vi "Get Mac address.vi"(8 "error in (no error)":errorcluster) -> (0 "error out":errorcluster, 3 "MAC address":string)   [LabVIEW 2016]
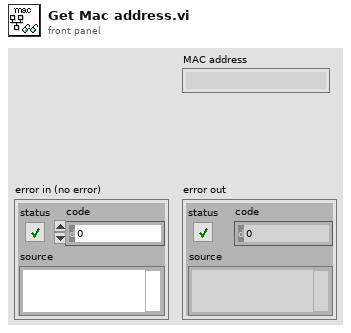
[diagram p1: front panel]
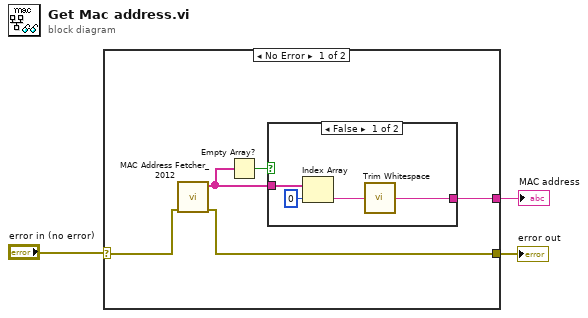
[diagram p0: block diagram]
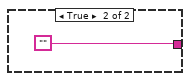
[diagram p2: hidden frame]
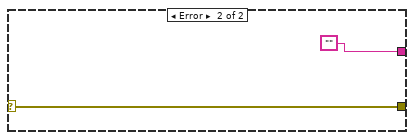
[diagram p3: hidden frame]
diagram:
  n1 = case shown="No Error" "error in (no error)" {
    selector: "error in (no error)" -> [w6 w15]
    tunnel: [w5 w15] -> w2
    tunnel: [w4 ""] -> w1
    frame No Error {
      n2 = call "MAC Address Fetcher_2012.vi"("error in (no error)"=w6) -> ("error out"=w5:errorcluster, "MAC Addresses"=w7:string[])  [unwired: 9 in]
      n3 = Empty Array?(array=w7) -> (empty?=w8:bool)
      n4 = case shown="False" w8 {
        tunnel: w7 -> [w12 _]
        tunnel: [w9 ""] -> w4
        frame False {
          n5 = Index Array(array=w12, index=0) -> (element=w10:string)
          n6 = call <vilib>:"Trim Whitespace.vi"("string"=w10) -> ("trimmed string"=w9:string)  [unwired: 1 in]
        }
        frame True {
        }
      }
    }
    frame Error {
    }
  }
  "error out" <- w2
  "MAC address" <- w1
